vi "Initiate.vi"(7 "If Empty":string="Cluster", 8 "error in (no error)":errorcluster, 10 "Prefix":string, 11 "Raw Variant":variant) -> (0 "error out":errorcluster, 3 "ClusterTree out":refnum<class "TreeLUT.lvclass">)   [LabVIEW 2017, in "TreeLUT.lvclass"]
uses:
  TreeLUT.lvclass
  ClusterTree.ctl
  <vilib>/Utility/Data Type/Type Definitions/Data Type.ctl
  TreeLUT.lvclass/TreeLUT.ctl
  <vilib>/Utility/Data Type/NI_Data Type.lvlib
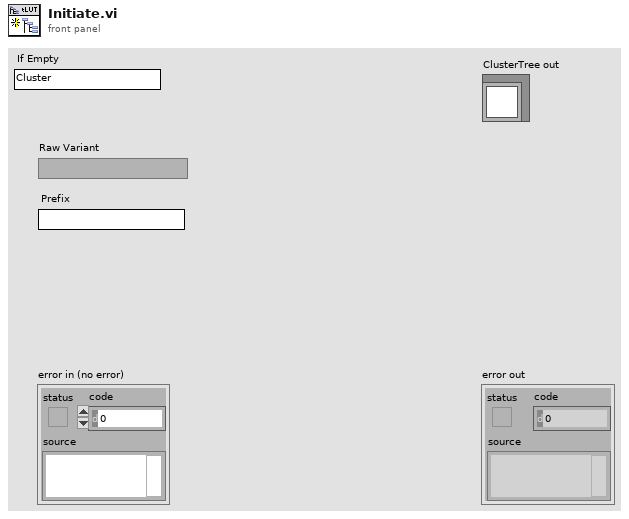
[diagram p1: front panel]
types:
  T1 = typedef "TreeLUT.lvclass/ClusterTree.ctl" = cluster{"LUT":variant, "Fields[]":string[], "ColHdrs[]":string[], "DataTypes[]":T2[], "Indents[]":i32[], "DataType LUT":variant}
  T2 = typedef "NI_Data Type.lvlib/Data Type.ctl" = enum8{"Invalid Type", "Void", "I8", "I16", "I32", "I64", "U8", "U16", "U32", "U64", "Single Float", "Double Float", "Extended Float", "Single Complex", "Double Complex", "Extended Complex", "Enum U8", "Enum U16", "Enum U32", "Enum U64", "Single Float With Unit", "Double Float With Unit", "Extended Float With Unit", "Single Complex with Unit", "Double Complex with Unit", "Extended Complex with Unit", "Boolean", "String", "Path", "Picture", "Tag", "Array", "Cluster", "Variant", "LV Variant", "Waveform", "Timestamp", "Digital Waveform", "Digital Data", "ExpressData", "Refnum", "External Data", "VI", "Poly VI", "LabVIEW Class Instance", "Fixed Point"}
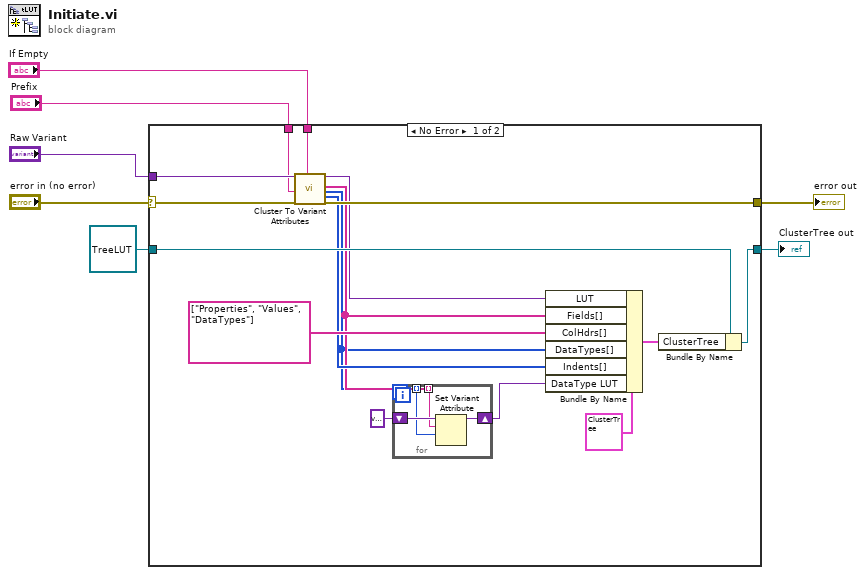
[diagram p0: block diagram]
diagram:
  n1 = case shown="No Error" "error in (no error)" {
    selector: "error in (no error)" -> [w20 w29]
    tunnel: [w19 w29] -> w6
    tunnel: [w22 w28] -> w4
    tunnel: refnum<class "TreeLUT.lvclass"> refnum ("ClusterTree in") -> [w23 w28]
    tunnel: "Raw Variant" -> [w21 _]
    tunnel: "Prefix" -> [w13 _]
    tunnel: "If Empty" -> [w12 _]
    frame No Error {
      n2 = call "Cluster To Variant Attributes.vi"("Variant of Cluster"=w21, "Prefix"=w13, "error in (no error)"=w20, "If Empty"=w12) -> ("Variant Attributes Out"=w15:variant, "Fields"=w10:string[], "DataTypes"=w9:T2[], "Indents"=w16:i32[], "error out"=w19:errorcluster)  [unwired: 11 in]
      n3 = for {
        shift-right: [w24] -> w8
        shift-left: variant -> [w27]
        tunnel: w10 -> [w26] mode=indexing
        tunnel: w9 -> [w25] mode=indexing
        n4 = Set Variant Attribute(Variant=w27, name=w26, value=w25) -> (Variant out=w24:variant)  [unwired: 1 in, 2 out]
      }
      n5 = Bundle By Name(cluster=T1 {"LUT"=variant, "Fields[]"=[], "ColHdrs[]"=[], "DataTypes[]"=[], "Indents[]"=[], "DataType LUT"=variant} ("ClusterTree"), "LUT"=w15, "Fields[]"=w10, "ColHdrs[]"=string[] ["Properties", "Values", "DataTypes"], "DataTypes[]"=w9, "Indents[]"=w16, "DataType LUT"=w8) -> (w18:T1)
      n6 = Bundle By Name(cluster=w23, "ClusterTree"=w18) -> (w22:refnum<class "TreeLUT.lvclass">)
    }
    frame Error {
    }
  }
  "error out" <- w6
  "ClusterTree out" <- w4
